vi "Sensor Data (Multiple Readings).vi"(6 "Reading Interval (100)":dbl=100.0, 7 "Sample Count (1)":i32=1, 8 "error in (no error)":errorcluster, 9 "Data Source (0:Kelvin)":u16(ring) items=["Kelvin", "Celsius", "Sensor Units"], 10 "Input (0:A)":u16(ring) items=["A", "B", "C", "D"], 11 "VISA resource name":refnum<visa-resource-name>) -> (0 "error out":errorcluster, 2 "Sensor Data":dbl[](array[numeric]) format="%.4f", 3 "VISA resource name out":refnum<visa-resource-name>)   [LabVIEW 2020, in "Lake Shore 336.lvlib"]
doc: "Reads and returns multiple sensor readings from the instrument. Control over interval between readings is also provided."
uses:
  Lake Shore 336.lvlib
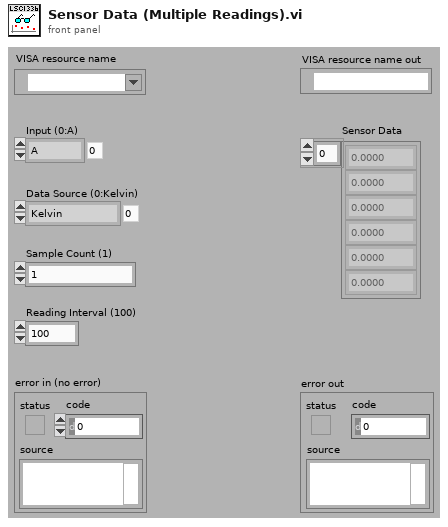
[diagram p1: front panel]
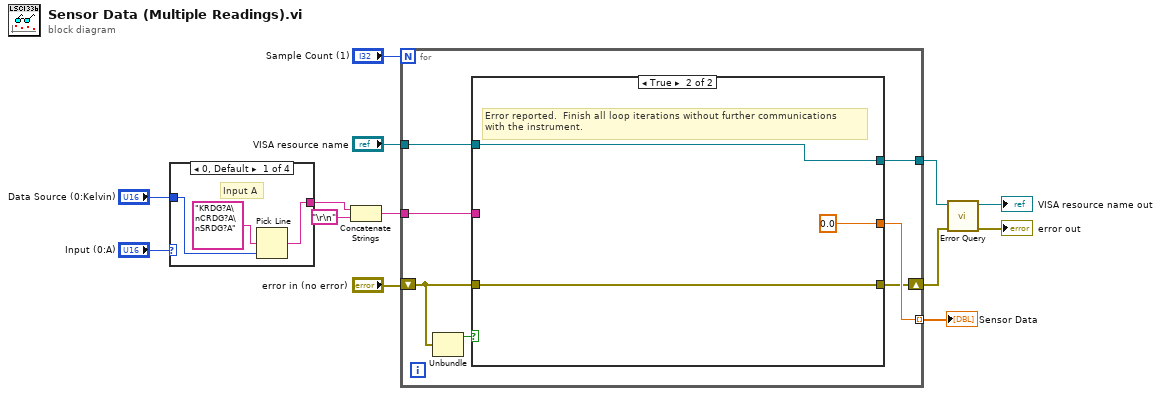
[diagram p0: block diagram]
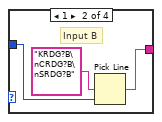
[diagram p2: hidden frame]
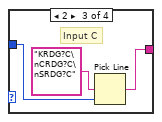
[diagram p3: hidden frame]
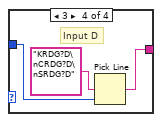
[diagram p4: hidden frame]
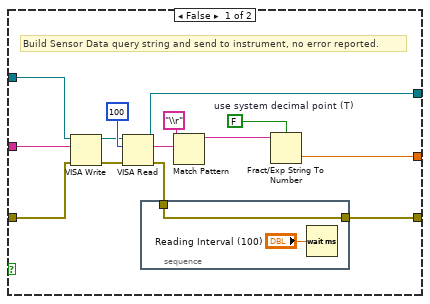
[diagram p5: hidden frame]
diagram:
  n1 = case shown="0, Default" "Input (0:A)" {
    tunnel: "Data Source (0:Kelvin)" -> [w15 w17 w20 w23]
    tunnel: [w14 w18 w21 w24] -> w4
    frame 0, Default {
      # "Input A"
      n2 = Pick Line(multi-line string="KRDG?A\nCRDG?A\nSRDG?A", line index=w15) -> (output string=w14:string)  [unwired: 1 in]
    }
    frame 1 {
      # "Input B"
      n3 = Pick Line(multi-line string="KRDG?B\nCRDG?B\nSRDG?B", line index=w17) -> (output string=w18:string)  [unwired: 1 in]
    }
    frame 2 {
      # "Input C"
      n4 = Pick Line(multi-line string="KRDG?C\nCRDG?C\nSRDG?C", line index=w20) -> (output string=w21:string)  [unwired: 1 in]
    }
    frame 3 {
      # "Input D"
      n5 = Pick Line(multi-line string="KRDG?D\nCRDG?D\nSRDG?D", line index=w23) -> (output string=w24:string)  [unwired: 1 in]
    }
  }
  n6 = Concatenate Strings(w4, "\r\n") -> (w3:string)
  n7 = for {
    N: "Sample Count (1)" -> [_]
    tunnel: "VISA resource name" -> [w32]
    tunnel: [w31] -> w10
    tunnel: w3 -> [w30]
    tunnel: [w29] -> w8 mode=indexing
    shift-right: [w28] -> w6
    shift-left: "error in (no error)" -> [w27]
    n8 = Unbundle(w27) -> ("status"=w26:bool)  [unwired: 2 out]
    n9 = case shown="True" w26 {
      tunnel: w32 -> [w46 w51]
      tunnel: [w45 w51] -> w31
      tunnel: w30 -> [w37 _]
      tunnel: [w36 0.0] -> w29
      tunnel: w27 -> [w35 w50]
      tunnel: [w33 w50] -> w28
      frame False {
        w39 = FALSE  # use system decimal point (T)
        # "Build Sensor Data query string and send to instrument, no error reported."
        n10 = VISA Write(VISA resource name=w46, write buffer=w37, error in (no error)=w35) -> (VISA resource name out=w41:refnum<visa-resource-name>, error out=w40:errorcluster)  [unwired: 1 out]
        n11 = VISA Read(VISA resource name=w41, byte count=100, error in (no error)=w40) -> (VISA resource name out=w45:refnum<visa-resource-name>, read buffer=w43:string, error out=w34:errorcluster)  [unwired: 1 out]
        n12 = stacked-sequence {
          tunnel: w34 -> [w47]
          tunnel: [w47] -> w33
          frame #0 {
            n13 = Wait (ms)(milliseconds to wait="Reading Interval (100)") -> ()  [unwired: 1 out]
          }
        }
        n14 = Match Pattern(string=w43, regular expression="\\r") -> (before substring=w38:string)  [unwired: 1 in, 3 out]
        n15 = Fract/Exp String To Number(use system decimal point (T)=w39, string=w38) -> (number=w36:dbl)  [unwired: 2 in, 1 out]
      }
      frame True {
        # "Error reported.  Finish all loop iterations without further communications\nwith the instrument."
      }
    }
  }
  "Sensor Data" <- w8
  n16 = call "Error Query.vi"("error in (no error)"=w6, "VISA resource name"=w10) -> ("error out"=→"error out":errorcluster, "VISA resource name out"=→"VISA resource name out":refnum<visa-resource-name>)  [unwired: 7 in, 1 out]
